vi "TETS Read Write.vi"(0 "Input Bytes":u8[](array[numeric]) format="%.0b", 2 "Timeout (ms)":i32=10000, 11 "error in":errorcluster) -> (4 "Output Bytes":u8[](array[numeric]) format="%.0b", 15 "error in":errorcluster)   [LabVIEW 2010]
uses:
  <instrlib>/Agilent 33XXX Series/Public/Configure/Configure Modulation (Amplitude).vi
  <instrlib>/Agilent 33XXX Series/Agilent 33XXX Series.lvlib
panel:
  out "Array":dbl[](array[numeric])
  out "error out":errorcluster
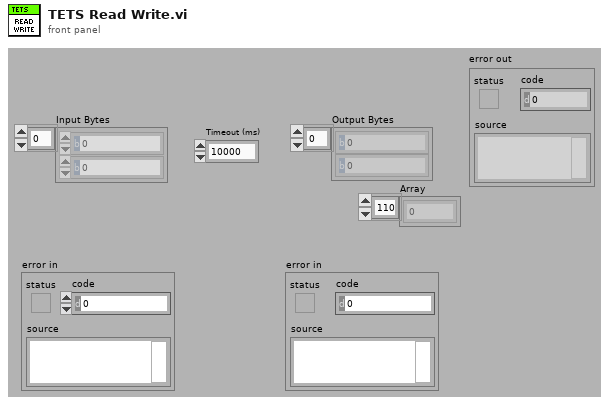
[diagram p1: front panel]
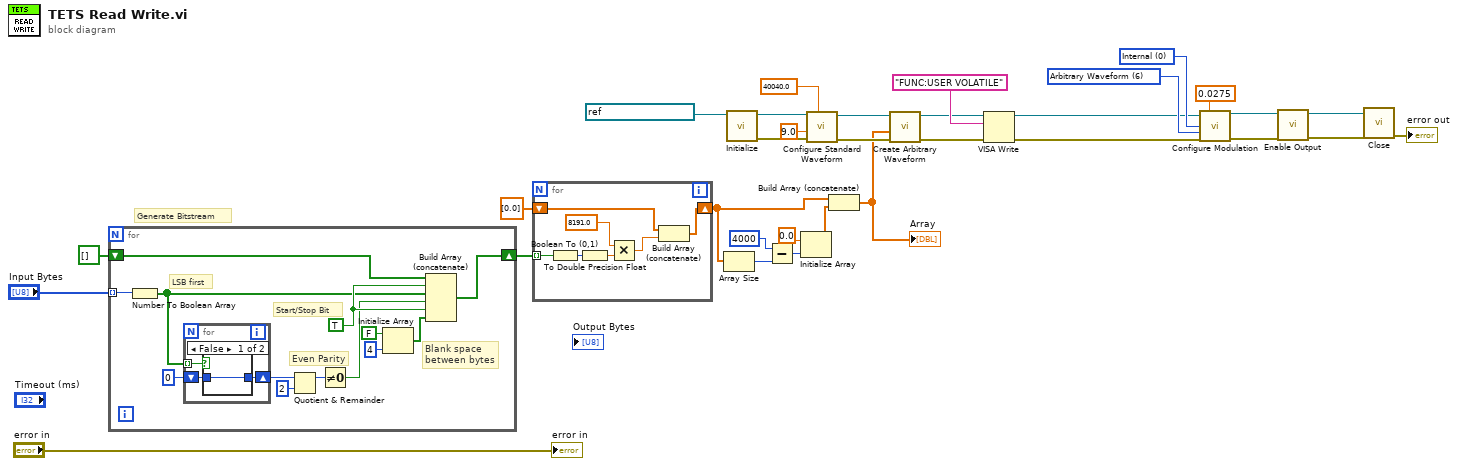
[diagram p0: block diagram]
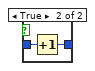
[diagram p2: hidden frame]
diagram:
  w19 = 6 items=["Sine", "Square", "Ramp", "Negative Ramp", "Triangle", "Noise", "Arbitrary Waveform"] ("Modulation Waveform (0: Sine)")
  w20 = 0 items=["Internal", "External"] ("AM Source (0: Internal)")
  # "Generate Bitstream"
  n1 = for {
    tunnel: "Input Bytes" -> [w45] mode=indexing
    shift-right: [w37] -> w29
    shift-left: bool[] [] -> [w36]
    w44 = TRUE
    # "LSB first"
    # "Blank space\nbetween bytes"
    # "Start/Stop Bit"
    # "Even Parity"
    n2 = Number To Boolean Array(number=w45) -> (Boolean array=w38:bool[])
    n3 = for {
      tunnel: w38 -> [w48] mode=indexing
      shift-right: [w46] -> w42
      shift-left: u8 0 -> [w47]
      n4 = case shown="False" w48 {
        tunnel: w47 -> [w49 w51]
        tunnel: [w49 w50] -> w46
        frame False {
        }
        frame True {
          n5 = Increment(x=w51) -> (x+1=w50:u8)
        }
      }
    }
    n6 = Quotient & Remainder(x=w42, y=u8 2) -> (x-y*floor(x/y)=w40:u8)  [unwired: 1 out]
    n7 = Not Equal To 0?(x=w40) -> (x != 0?=w39:bool)
    n8 = Initialize Array(FALSE, 4 ("dimension size")) -> (w33:bool[])
    n9 = Build Array (concatenate)(w36, w44, w38, w39, w44, w33) -> (w37:bool[])
  }
  n10 = for {
    tunnel: w29 -> [w58] mode=indexing
    shift-right: [w54] -> w7
    shift-left: dbl[] [0.0] -> [w53]
    n11 = Boolean To (0,1)(Boolean=w58) -> (0, 1=w57:i16)
    n12 = To Double Precision Float(number=w57) -> (double precision float=w56:dbl)
    n13 = Multiply(x=8191.0, y=w56) -> (x*y=w52:dbl)
    n14 = Build Array (concatenate)(w53, w52) -> (w54:dbl[])
  }
  n15 = Array Size(array=w7) -> (size(s)=w12:i32)
  n16 = call <instrlib>:"Initialize.vi"("VISA resource name"=refnum<visa-resource-name> "GPIB0::7::INSTR") -> ("error out"=w27:errorcluster, "VISA resource name out"=w28:refnum<visa-resource-name>)  [unwired: 9 in]
  n17 = Subtract(x=4000, y=w12) -> (x-y=w10:i32)
  n18 = Initialize Array(0.0, w10) -> (w8:dbl[])
  n19 = call <instrlib>:"Configure Standard Waveform.vi"("Frequency (1000 Hz)"=40040.0, "error in (no error)"=w27, "Amplitude (1)"=9.0, "VISA resource name"=w28) -> ("error out"=w23:errorcluster, "VISA resource name out"=w24:refnum<visa-resource-name>)  [unwired: 6 in]
  n20 = Build Array (concatenate)(w7, w8) -> (w6:dbl[])
  "Array" <- w6
  n21 = call <instrlib>:"Create Arbitrary Waveform.vi"("error in (no error)"=w23, "Arbitrary Waveform Data"=w6, "VISA resource name"=w24) -> ("error out"=w2:errorcluster, "VISA resource name out"=w4:refnum<visa-resource-name>)  [unwired: 7 in]
  n22 = VISA Write(VISA resource name=w4, write buffer="FUNC:USER VOLATILE" ("true string"), error in (no error)=w2) -> (VISA resource name out=w3:refnum<visa-resource-name>, error out=w1:errorcluster)  [unwired: 1 out]
  n23 = call-poly <instrlib>:"Configure Modulation.vi"("VISA resource name"=w3, "Modulation Frequency (1000 Hz)"=0.0275 ("Frequency (1000 Hz)"), "AM Source (0: Internal)"=w20, "Modulation Waveform (0: Sine)"=w19, "error in (no error)"=w1) -> ("VISA resource name out"=w18:refnum<visa-resource-name>, "error out"=w17:errorcluster)  [unwired: 9 in]
  n24 = call <instrlib>:"Enable Output.vi"("error in (no error)"=w17, "VISA resource name"=w18) -> ("error out"=w15:errorcluster, "VISA resource name out"=w16:refnum<visa-resource-name>)  [unwired: 8 in]
  n25 = call <instrlib>:"Close.vi"("error in (no error)"=w15, "VISA resource name"=w16) -> ("error out"=→"error out":errorcluster)  [unwired: 9 in]
  "error in" <- "error in"
